vi "Word to bytes.vi"(5 "Litt/BigEnd":bool, 7 "Index":i32, 8 "Word":u16, 9 "Image Data in":u8[](array[numeric])) -> (1 "Index+2":i32, 3 "Image Data out":u8[](array[numeric]))   [LabVIEW 2015, in "Tiff reader.lvlib"]
doc: "This .vi converts word to 2bytes."
uses:
  Tiff reader.lvlib
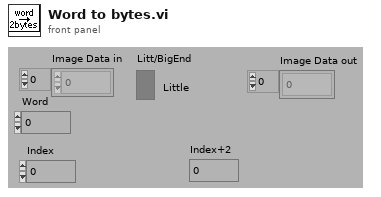
[diagram p1: front panel]
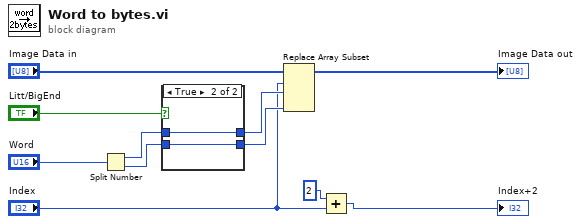
[diagram p0: block diagram]
diagram:
  n1 = Split Number(x="Word") -> (hi(x)=w9:u8, lo(x)=w8:u8)
  n2 = case shown="True" "Litt/BigEnd" {
    tunnel: [w12 w15] -> w6
    tunnel: w9 -> [w13 w15]
    tunnel: [w13 w14] -> w5
    tunnel: w8 -> [w12 w14]
    frame False {
    }
    frame True {
    }
  }
  n3 = Replace Array Subset "Replace Array Subset"(array="Image Data in", new element #1=w6, index #1="Index", new element #2=w5) -> (→"Image Data out":u8[])  [unwired: 1 in]
  n4 = Add(x=2, y="Index") -> (x+y=→"Index+2":i32)
